vi "Assinante2.vi"() -> ()   [LabVIEW 2018]
uses:
  RxTx/CM_RxTx.lvclass
  <vilib>/addons/zeromq/zmq_context.lvclass
  socket REQ/socket REQ.lvclass
  C:/Users/Denis/Desktop/communication-manager/communication-manager/Socket/Socket.lvclass
  socket SUB/socket SUB.lvclass
  Socket/Socket.lvclass
panel:
  in  "socket SUB.lvclass":refnum<class "socket SUB.lvclass">
  in  "socket REQ.lvclass":refnum<class "socket REQ.lvclass">
  out "error out":errorcluster
  out "context":refnum<class "zmq_context.lvclass">
  in  "Queue TX":refnum<class "CM_RxTx.lvclass">
  in  "Queue RX":refnum<class "CM_RxTx.lvclass">
  out "reply":string
  in  "Comm Type":string(combo)="REQ"
  in  "publication":string
  in  "send":bool
  in  "stop":bool
  # "REQ/SUB endpoint"
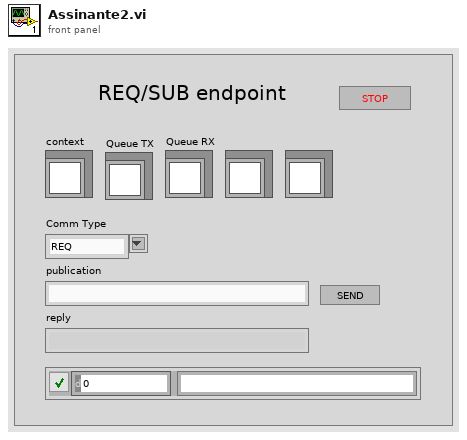
[diagram p1: front panel]
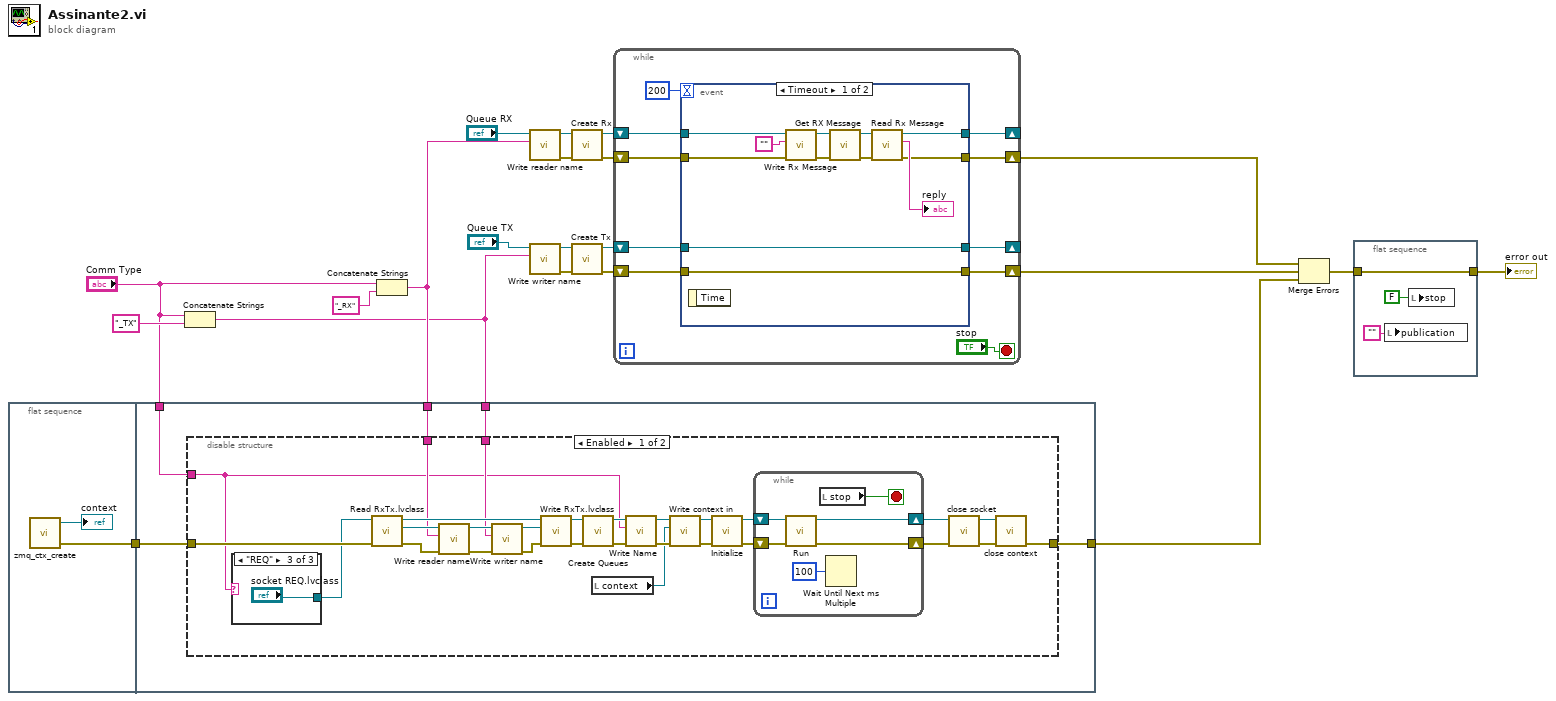
[diagram p0: block diagram]
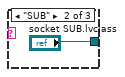
[diagram p3: hidden frame]
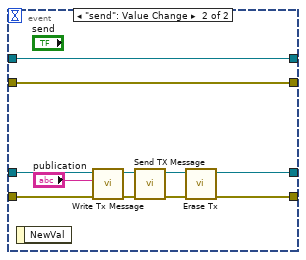
[diagram p5: hidden frame]
diagram:
  n1 = flat-sequence {
    tunnel: [w22] -> w7
    tunnel: [w28] -> w8
    tunnel: w7 -> [w27]
    tunnel: w3 -> [w26]
    tunnel: w2 -> [w25]
    tunnel: "Comm Type" -> [w24]
    frame #0 {
      n2 = call <vilib>:"zmq_ctx_create.vi"() -> ("error out"=w22:errorcluster, "context out"=→"context":refnum<class "zmq_context.lvclass">)  [unwired: 4 in]
    }
    frame #1 {
      n3 = disable-structure shown="Enabled" {
        disable-tunnel: [w34 _] -> w28
        disable-tunnel: w27 -> [w33 _]
        disable-tunnel: w26 -> [w32 _]
        disable-tunnel: w25 -> [w31 _]
        disable-tunnel: w24 -> [w30 _]
        frame Enabled {
          n4 = case shown="\"REQ\"" w30 {
            tunnel: [_ "socket SUB.lvclass" "socket REQ.lvclass"] -> w29
            frame "False", Default {
            }
            frame "SUB" {
            }
            frame "REQ" {
            }
          }
          n5 = call-dynamic "Read RxTx.lvclass.vi"("error in (no error)"=w33, "Socket in"=w29) -> ("error out"=w50:errorcluster, "RxTx.lvclass"=w56:refnum<class "CM_RxTx.lvclass">, "Socket out"=w53:refnum<class "Socket.lvclass">)  [unwired: 7 in]
          n6 = call-dynamic "Write reader name.vi"("error in (no error)"=w50, "RX name"=w32, "RxTx in"=w56) -> ("error out"=w49:errorcluster, "RxTx out"=w55:refnum<class "CM_RxTx.lvclass">)  [unwired: 7 in]
          n7 = call-dynamic "Write writer name.vi"("error in (no error)"=w49, "Tx name"=w31, "RxTx in"=w55) -> ("error out"=w48:errorcluster, "RxTx out"=w54:refnum<class "CM_RxTx.lvclass">)  [unwired: 7 in]
          n8 = call-dynamic "Write RxTx.lvclass.vi"("error in (no error)"=w48, "RxTx.lvclass"=w54, "Socket in"=w53) -> ("error out"=w51:errorcluster, "Socket out"=w52:refnum<class "Socket.lvclass">)  [unwired: 7 in]
          n9 = call-dynamic "Create Queues.vi"("error in (no error)"=w51, "Socket in"=w52) -> ("error out"=w44:errorcluster, "Socket out"=w47:refnum<class "Socket.lvclass">)  [unwired: 8 in]
          n10 = local read "context"() -> (w37:refnum<class "zmq_context.lvclass">)
          n11 = call-dynamic "Write Name.vi"("error in (no error)"=w44, "Name"=w30, "Socket in"=w47) -> ("error out"=w43:errorcluster, "Socket out"=w46:refnum<class "Socket.lvclass">)  [unwired: 7 in]
          n12 = call-dynamic "Write context in.vi"("error in (no error)"=w43, "zeromq.lvlib:ZeroMQ Context"=w37, "Socket in"=w46) -> ("error out"=w42:errorcluster, "Socket out"=w45:refnum<class "Socket.lvclass">)  [unwired: 7 in]
          n13 = call-dynamic "Initialize.vi"("error in (no error)"=w42, "Socket in"=w45) -> ("error out"=w39:errorcluster, "Socket out"=w41:refnum<class "Socket.lvclass">)  [unwired: 8 in]
          n14 = while {
            shift-right: [w63] -> w40
            shift-left: w41 -> [w64]
            shift-right: [w61] -> w38
            shift-left: w39 -> [w62]
            stop <- w59 stop-if-true
            n15 = call-dynamic "Run.vi"("error in (no error)"=w62, "Socket in"=w64) -> ("error out"=w61:errorcluster, "Socket out"=w63:refnum<class "Socket.lvclass">)  [unwired: 8 in]
            n16 = local read "stop"() -> (w59:bool)
            n17 = Wait Until Next ms Multiple(millisecond multiple=u32 100) -> ()  [unwired: 1 out]
          }
          n18 = call "close socket.vi"("error in (no error)"=w38, "Socket in"=w40) -> ("error out"=w36:errorcluster, "Socket out"=w35:refnum<class "Socket.lvclass">)  [unwired: 8 in]
          n19 = call-dynamic "close context.vi"("error in (no error)"=w36, "Socket in"=w35) -> ("error out"=w34:errorcluster)  [unwired: 8 in, 1 out]
        }
        frame Disabled {
        }
      }
    }
  }
  n20 = Concatenate Strings("Comm Type", "_TX" ("string")) -> (w2:string)
  n21 = Concatenate Strings("Comm Type", "_RX" ("string")) -> (w3:string)
  n22 = call-dynamic "Write reader name.vi"("RX name"=w3, "RxTx in"="Queue RX") -> ("error out"=w15:errorcluster, "RxTx out"=w16:refnum<class "CM_RxTx.lvclass">)  [unwired: 8 in]
  n23 = call-dynamic "Write writer name.vi"("Tx name"=w2, "RxTx in"="Queue TX") -> ("error out"=w13:errorcluster, "RxTx out"=w17:refnum<class "CM_RxTx.lvclass">)  [unwired: 8 in]
  n24 = call "Create Rx.vi"("error in (no error)"=w15, "RxTx in"=w16) -> ("error out"=w11:errorcluster, "RxTx out"=w19:refnum<class "CM_RxTx.lvclass">)  [unwired: 8 in]
  n25 = call "Create Tx.vi"("error in (no error)"=w13, "RxTx in"=w17) -> ("error out"=w12:errorcluster, "RxTx out"=w21:refnum<class "CM_RxTx.lvclass">)  [unwired: 8 in]
  n26 = while {
    shift-right: [w73] -> _
    shift-left: w21 -> [w74]
    shift-right: [w69] -> _
    shift-left: w19 -> [w70]
    shift-right: [w67] -> w9
    shift-left: w12 -> [w68]
    shift-right: [w65] -> w10
    shift-left: w11 -> [w66]
    stop <- "stop" stop-if-true
    n27 = event shown="[0] Timeout" {
      selector: _ -> [_ _]
      dyn-events: _ -> [_ _]
      timeout: 200 -> [_ _]
      tunnel: w74 -> [w86 w97]
      tunnel: [w86 w87] -> w73
      tunnel: w70 -> [w82 w93]
      tunnel: [w80 w93] -> w69
      tunnel: w68 -> [w77 w92]
      tunnel: [w77 w88] -> w67
      tunnel: w66 -> [w76 w91]
      tunnel: [w75 w91] -> w65
      event Timeout {
        n28 = event-data() -> ()  [unwired: 1 in, 1 out]
        n29 = call "Write Rx Message.vi"("error in (no error)"=w76, "Rx Message"="", "RxTx in"=w82) -> ("error out"=w79:errorcluster, "RxTx out"=w81:refnum<class "CM_RxTx.lvclass">)  [unwired: 7 in]
        n30 = call "Get RX Message.vi"("error in (no error)"=w79, "RxTx in"=w81) -> ("error out"=w83:errorcluster, "RxTx out"=w85:refnum<class "CM_RxTx.lvclass">)  [unwired: 7 in, 1 out]
        n31 = call "Read Rx Message.vi"("error in (no error)"=w83, "RxTx in"=w85) -> ("error out"=w75:errorcluster, "Rx Message"=→"reply":string, "RxTx out"=w80:refnum<class "CM_RxTx.lvclass">)  [unwired: 7 in]
      }
      event "send": Value Change {
        n32 = event-data() -> ()  [unwired: 1 in, 1 out]
        n33 = call "Write Tx Message.vi"("error in (no error)"=w92, "Tx Message"="publication", "RxTx in"=w97) -> ("error out"=w94:errorcluster, "RxTx out"=w95:refnum<class "CM_RxTx.lvclass">)  [unwired: 7 in]
        n34 = call "Send TX Message.vi"("error in (no error)"=w94, "RxTx in"=w95) -> ("error out"=w89:errorcluster, "RxTx out"=w90:refnum<class "CM_RxTx.lvclass">)  [unwired: 8 in]
        n35 = call "Erase Tx.vi"("error in (no error)"=w89, "RxTx in"=w90) -> ("error out"=w88:errorcluster, "RxTx out"=w87:refnum<class "CM_RxTx.lvclass">)  [unwired: 8 in]
      }
    }
  }
  n36 = Merge Errors(w10, w9, w8) -> (w5:errorcluster)
  n37 = flat-sequence {
    tunnel: w5 -> [w100]
    tunnel: [w100] -> w4
    frame #0 {
      n38 = local write "publication"("") -> ()
      n39 = local write "stop"(FALSE ("stop")) -> ()
    }
  }
  "error out" <- w4
